vi "Set Data Logging Rate (Custom Rate).vi"(8 "error in (no error)":errorcluster, 10 "Custom Rate (Hz)":dbl, 11 "Data Logging Specification Ref in":T1) -> (0 "error out":errorcluster, 3 "Data Logging Specification Ref out":T1)   [LabVIEW 2020, in "NI_VS Data Logging API.lvlib"]
doc: "Specifies the rate at which to log data, in hertz. You can log at the rate at which the target produces data, or a custom rate. You must manually select the polymorphic instance to use."
uses:
  <vilib>/NI VeriStand/Execution/DataLogging/NI_VS Data Logging API.lvlib
  <vilib>/NI VeriStand/Execution/DataLogging/DataLoggingSpecification Ref.ctl
  NationalInstruments.VeriStand.ClientAPI
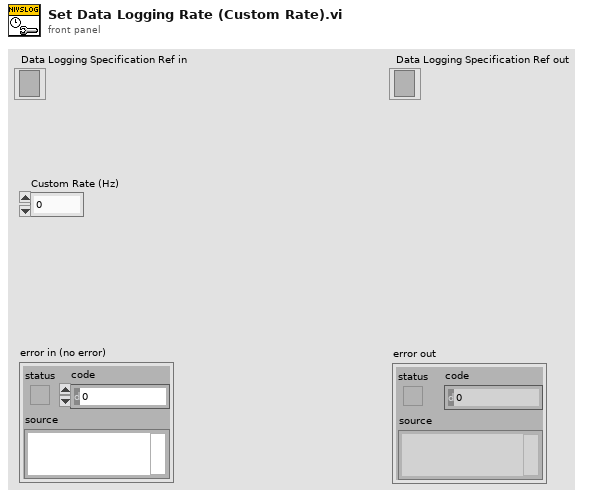
[diagram p1: front panel]
types:
  T1 = typedef "NI_VS Data Logging API.lvlib/DataLoggingSpecification Ref.ctl" = refnum<k24>
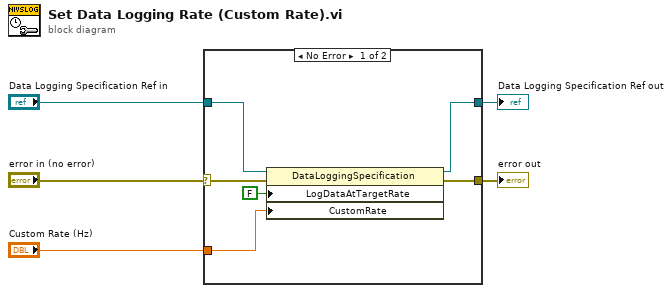
[diagram p0: block diagram]
diagram:
  n1 = case shown="No Error" "error in (no error)" {
    selector: "error in (no error)" -> [w11 w12]
    tunnel: "Data Logging Specification Ref in" -> [w10 w13]
    tunnel: [w9 w13] -> w3
    tunnel: [w8 w12] -> w2
    tunnel: "Custom Rate (Hz)" -> [w6 _]
    frame No Error {
      n2 = property class="DataLoggingSpecification"(reference=w10, error in=w11, "LogDataAtTargetRate"=FALSE, "CustomRate"=w6) -> (reference out=w9:T1, error out=w8:errorcluster)
    }
    frame Error {
    }
  }
  "error out" <- w2
  "Data Logging Specification Ref out" <- w3
